vi "Part 1.vi"(11 "Input":string) -> (3 "Output":i64)   [LabVIEW 2021]
panel:
  out "Map Out":string[][](array[string])
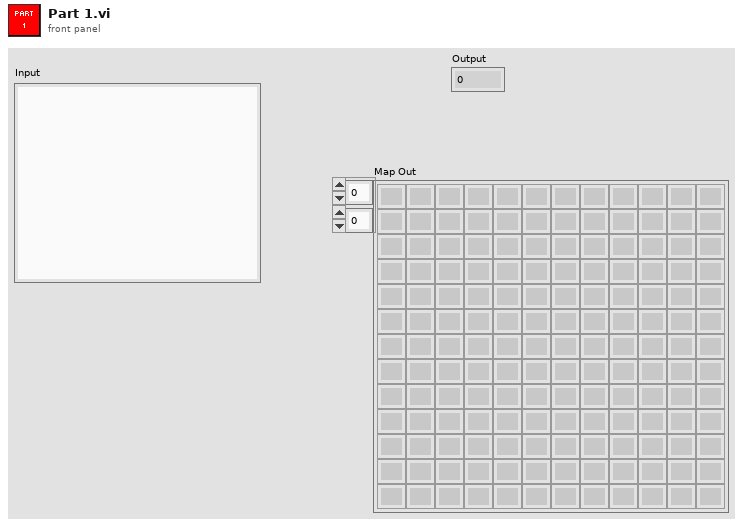
[diagram p1: front panel]
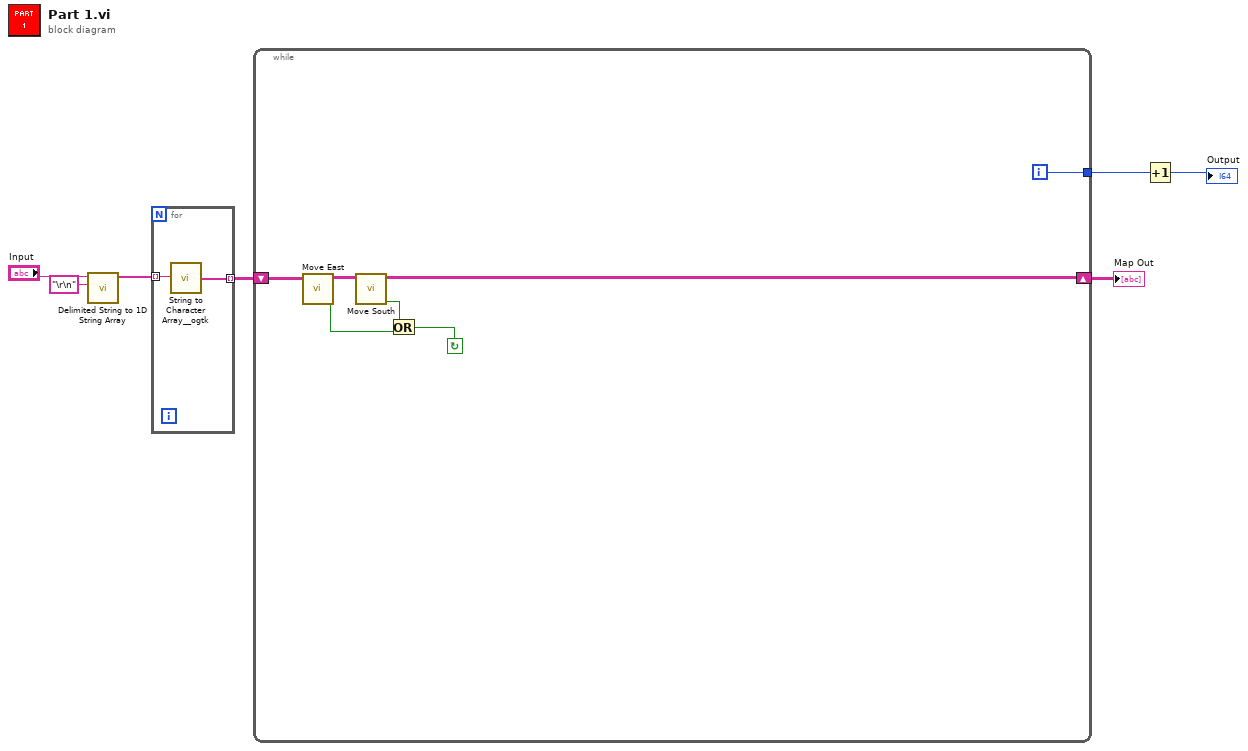
[diagram p0: block diagram]
diagram:
  n1 = call <vilib>:"Delimited String to 1D String Array.vi"("delimiter"="\r\n", "delimited string"="Input") -> ("string array"=w5:string[])  [unwired: 9 in]
  n2 = for {
    tunnel: w5 -> [w9] mode=indexing
    tunnel: [w8] -> w4 mode=indexing
    n3 = call <userlib>:"String to Character Array__ogtk.vi"("Input String"=w9) -> ("Character Array"=w8:string[])
  }
  n4 = while {
    shift-right: [w13] -> w3
    shift-left: w4 -> [w16]
    tunnel: [w15] -> w2
    i -> [w15]
    stop <- w11 continue-if-true
    n5 = call "Move East.vi"("Map In"=w16) -> ("Moved?"=w10:bool, "Map Out"=w14:string[][])  [unwired: 9 in]
    n6 = call "Move South.vi"("Map In"=w14) -> ("Moved?"=w12:bool, "Map Out"=w13:string[][])  [unwired: 9 in]
    n7 = Or(x=w12, y=w10) -> (x .or. y?=w11:bool)
  }
  "Map Out" <- w3
  n8 = Increment(x=w2) -> (x+1=→"Output":i32)
